vi "runtest client check.vi"(6 "Client IP or Domain Name (\"\")":string, 7 "POST (empty)":T4, 8 "error in (no error)":errorcluster, 9 "sxSequenceId":string, 10 "Username (\"\")":string, 11 "Connection Refnum":T5) -> (0 "error out":errorcluster, 3 "Connection Refnum":T5, 4 "User/Station":T1, 5 "POST out":T4)   [LabVIEW 2011]
uses:
  Summitek EXT/ODBC/SQL Controls/Connection Refnum.ctl
  ITK EXT/utils/keyedarr.llb/Keyed Array.ctl
  runtest User - Station.ctl
  server/database/Stations/Instruments/Instrument Record.ctl
  server/database/Stations/Step Associations/Step Association Record.ctl
  Summitek EXT/Miscellaneous/OGAB Version.ctl
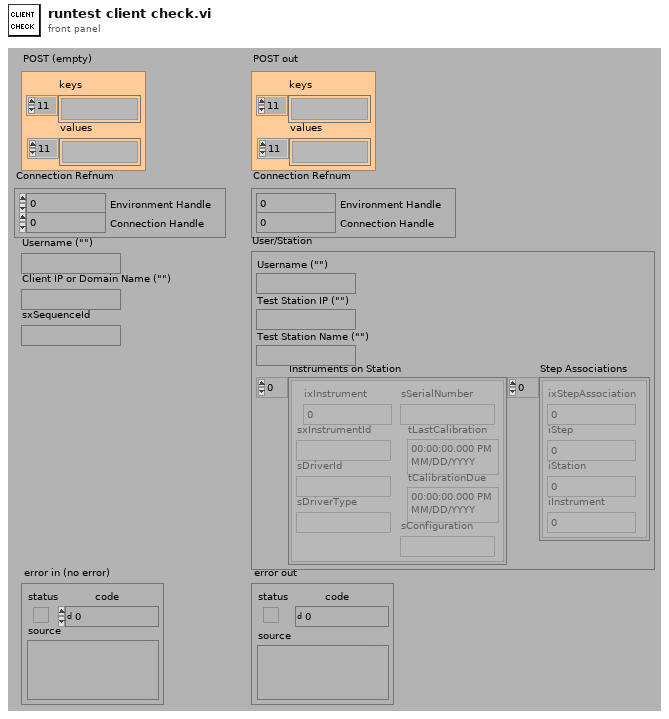
[diagram p1: front panel]
types:
  T1 = typedef "runtest User - Station.ctl" = cluster{"Username (\"\")":string, "Test Station IP (\"\")":string, "Test Station Name (\"\")":string, "Instruments on Station":T2[], "Step Associations":T3[]}
  T2 = typedef "Instrument Record.ctl" = cluster{"ixInstrument":i32, "sxInstrumentId":string, "sDriverId":string, "sDriverType":string, "sSerialNumber":string, "tLastCalibration":timestamp, "tCalibrationDue":timestamp, "sConfiguration":string}
  T3 = typedef "Step Association Record.ctl" = cluster{"ixStepAssociation":i32, "iStep":i32, "iStation":i32, "iInstrument":i32}
  T4 = typedef "Keyed Array.ctl" = cluster{"keys":string[], "values":string[]}
  T5 = typedef "Connection Refnum.ctl" = cluster{"Environment Handle":i32, "Connection Handle":i32}
  T6 = enum32{"invalid app kind", "Development System", "Run Time System", "Student Edition", "Embedded LabVIEW", "Evaluation", "Custom"}
  T7 = typedef "Station Record.ctl" = cluster{"ixStation":i32, "sxStationId":string, "sIP":string, "fVerified":bool}
  T8 = typedef "OGAB Version.ctl" = cluster{"Version":string, "Build Number":u32, "Build Date/Time":dbl}
  T9 = enum16{"Version 1 < Version 2", "Version 1 = Version 2", "Version 1 > Version 2"}
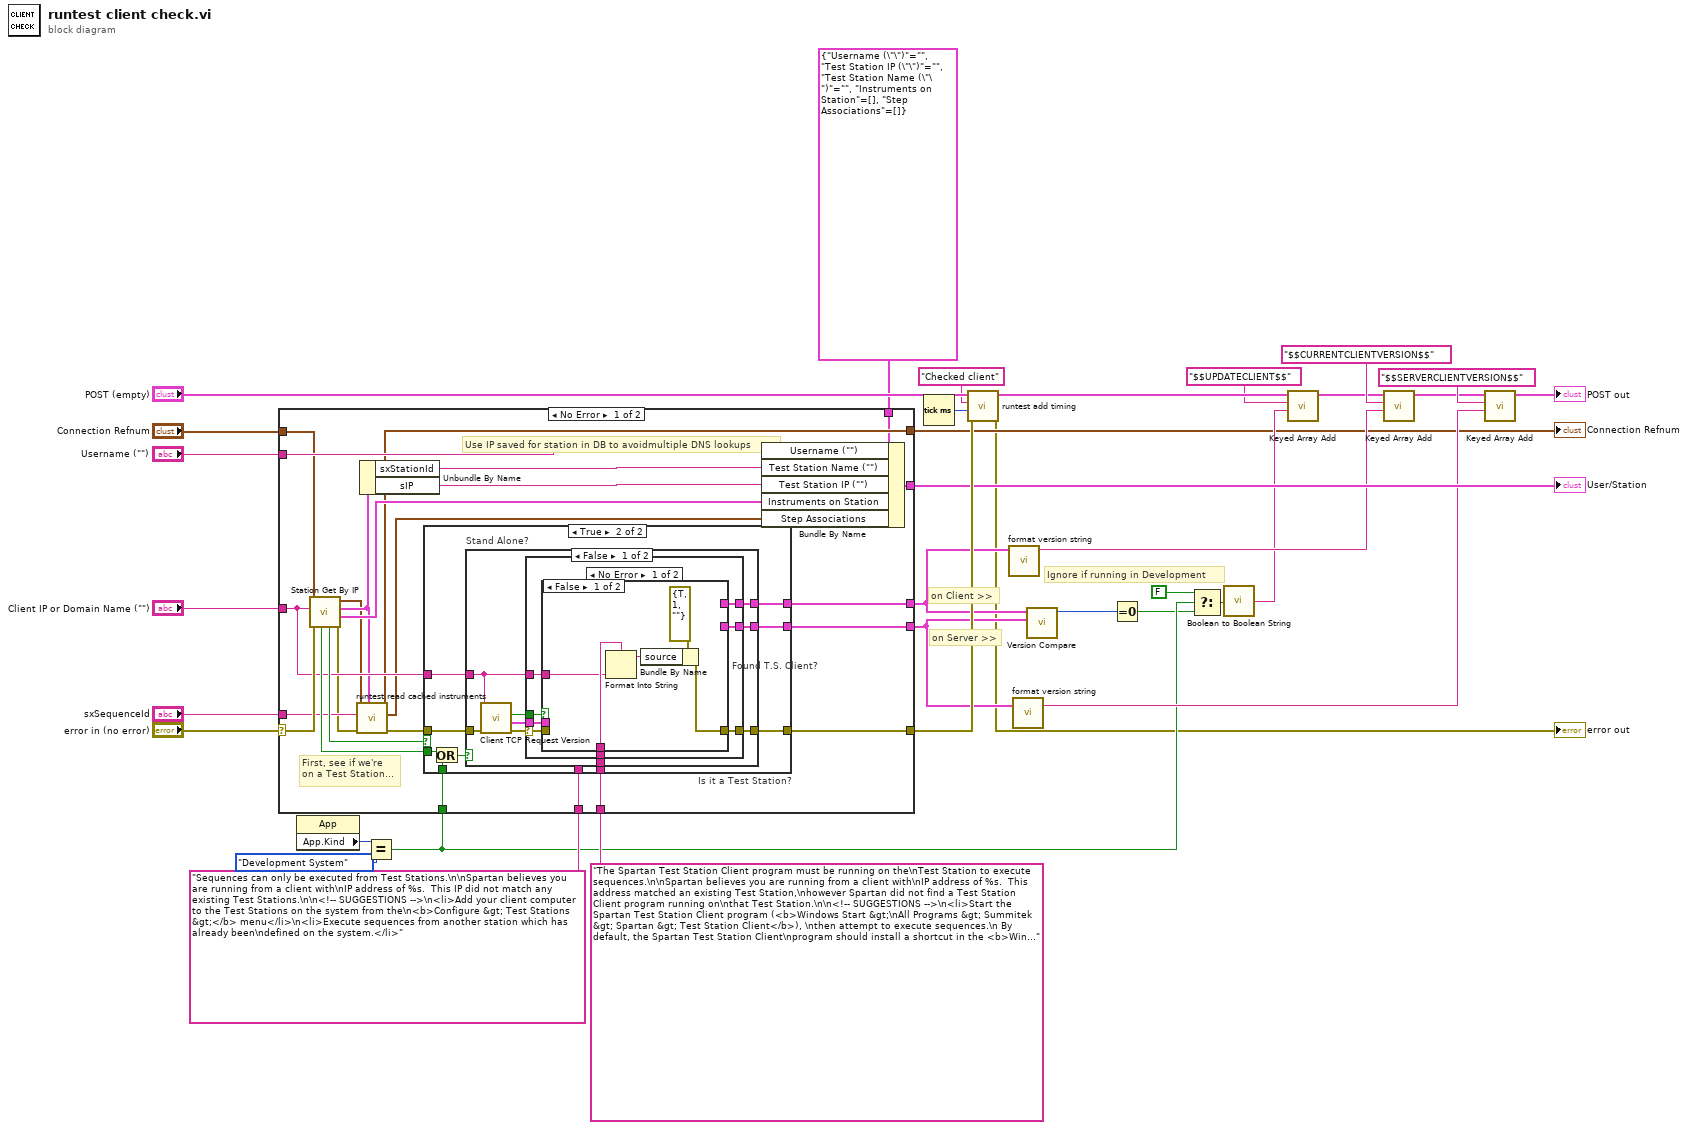
[diagram p0: block diagram]
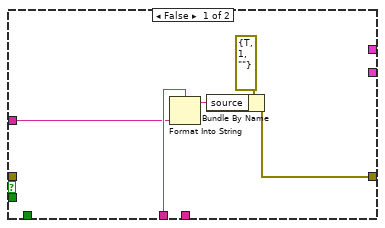
[diagram p2: hidden frame]
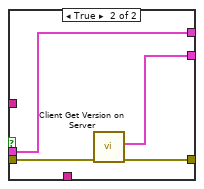
[diagram p3: hidden frame]
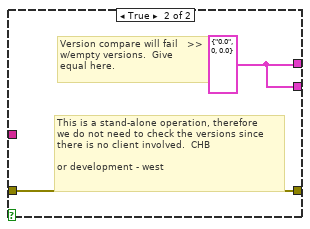
[diagram p5: hidden frame]
diagram:
  # "Ignore if running in Development"
  # "on Server >>"
  # "on Client >>"
  n1 = property class="App"() -> ("App.Kind"=w15:T6)  [unwired: 2 in, 2 out]
  n2 = Equal?(x=w15, y=T6."Development System") -> (x = y?=w11:bool)
  n3 = case shown="No Error" "error in (no error)" {
    selector: "error in (no error)" -> [w49 w103]
    tunnel: "Connection Refnum" -> [w48 w102]
    tunnel: [w39 w102] -> w4
    tunnel: "Client IP or Domain Name (\"\")" -> [w44 _]
    tunnel: [w58 w103] -> w28
    tunnel: "Sequences can only be executed from Test Stations.\n\nSpartan believes you are running from a client with\nIP address of %s.  This IP did not match any existing Test Stations.\n\n<!-- SUGGESTIONS -->\n<li>Add your client computer to the Test Stations on the system from the\n<b>Configure &gt; Test Stations &gt;</b> menu</li>\n<li>Execute sequences from another station which has already been\ndefined on the system.</li>" ("source") -> [w57 _]
    tunnel: "The Spartan Test Station Client program must be running on the\nTest Station to execute sequences.\n\nSpartan believes you are running from a client with\nIP address of %s.  This address matched an existing Test Station,\nhowever Spartan did not find a Test Station Client program running on\nthat Test Station.\n\n<!-- SUGGESTIONS -->\n<li>Start the Spartan Test Station Client program (<b>Windows Start &gt;\nAll Programs &gt; Summitek &gt; Spartan &gt; Test Station Client</b>), \nthen attempt to execute sequences.\n By default, the Spartan Test Station Client\nprogram should install a shortcut in the <b>Windows &gt; All Programs &gt;\nStartup</b> folder which would start the client automatically when you log in.</li>\n<li>By default Spartan uses TCP port 3363 to communicate with Test Station Clients.\nEnsure that this port is not blocked on either Spartan or the Client machine.</li>" ("source") -> [w56 _]
    tunnel: "Username (\"\")" -> [w55 _]
    tunnel: [w53 _] -> w26
    tunnel: [w52 _] -> w10
    tunnel: [w51 _] -> w9
    tunnel: w11 -> [w43 _]
    tunnel: "sxSequenceId" -> [w42 _]
    tunnel: T1 {"Username (\"\")"="", "Test Station IP (\"\")"="", "Test Station Name (\"\")"="", "Instruments on Station"=[], "Step Associations"=[]} ("User/Station") -> [w38 _]
    frame No Error {
      # "Use IP saved for station in DB to avoidmultiple DNS lookups"
      # "First, see if we're\non a Test Station..."
      n4 = call "Station Get By IP.vi"("error in (no error)"=w49, "IP or Name (\"\")"=w44, "Connection Refnum"=w48) -> ("error out"=w35:errorcluster, "Instruments on Station"=w47:T2[], "Station Record"=w41:T7, "Connection Refnum"=w40:T5, "Data Present?"=w45:bool, "Stand Alone?"=w46:bool)  [unwired: 1 in, 2 out]
      n5 = call "runtest read cached instruments.vi"("Station"=w41, "error in (no error)"=w35, "sxSequenceId"=w42, "Connection Refnum"=w40) -> ("error out"=w36:errorcluster, "Step Associations"=w37:T3[], "Connection Refnum"=w39:T5)  [unwired: 5 in]
      n6 = Unbundle By Name(w41) -> ("sxStationId"=w54:string, "sIP"=w50:string)
      n7 = case "Is it a Test Station?" shown="True" w45 {
        tunnel: w36 -> [_ w64]
        tunnel: w44 -> [w59 w65]
        tunnel: [w61 w72] -> w58
        tunnel: w57 -> [w63 _]
        tunnel: w56 -> [_ w71]
        tunnel: [_ w70] -> w52
        tunnel: [_ w69] -> w51
        tunnel: w46 -> [_ w67]
        tunnel: w43 -> [_ w68]
        frame False {
          n8 = Format Into String(format string=w63, w59) -> (resulting string=w60:string)  [unwired: 2 in, 1 out]
          n9 = Bundle By Name(cluster=errorcluster {"status"=TRUE, "code"=1, "source"=""} ("error out"), "source"=w60) -> (w61:errorcluster)
        }
        frame True {
          n10 = Or(x=w67, y=w68) -> (x .or. y?=w66:bool)
          n11 = case "Stand Alone?" shown="False" w66 {
            tunnel: w64 -> [w81 w101]
            tunnel: [w79 w101] -> w72
            tunnel: w71 -> [w78 _]
            tunnel: w65 -> [w77 _]
            tunnel: [w75 w100] -> w70
            tunnel: [w74 w100] -> w69
            frame False {
              n12 = call "Client TCP Request Version.vi"("error in (no error)"=w81, "Client IP"=w77) -> ("error out"=w73:errorcluster, "Client Version"=w76:T8, "Client Detected?"=w80:bool)  [unwired: 7 out]
              n13 = case shown="No Error" w73 {
                selector: w73 -> [w82 w99]
                tunnel: w80 -> [w89 _]
                tunnel: [w88 w99] -> w79
                tunnel: w78 -> [w87 _]
                tunnel: w77 -> [w86 _]
                tunnel: w76 -> [w85 _]
                tunnel: [w84 _] -> w75
                tunnel: [w83 _] -> w74
                frame No Error {
                  n14 = case "Found T.S. Client?" shown="False" w89 {
                    tunnel: w82 -> [_ w98]
                    tunnel: [w90 w97] -> w88
                    tunnel: w87 -> [w92 _]
                    tunnel: w86 -> [w91 _]
                    tunnel: w85 -> [_ w96]
                    tunnel: [_ w96] -> w84
                    tunnel: [_ w95] -> w83
                    frame False {
                      n15 = Format Into String(format string=w92, w91) -> (resulting string=w93:string)  [unwired: 2 in, 1 out]
                      n16 = Bundle By Name(cluster=errorcluster {"status"=TRUE, "code"=1, "source"=""} ("error out"), "source"=w93) -> (w90:errorcluster)
                    }
                    frame True {
                      n17 = call "Client Get Version on Server.vi"("error in (no error)"=w98) -> ("error out"=w97:errorcluster, "Version"=w95:T8)  [unwired: 9 out]
                    }
                  }
                }
                frame Error {
                }
              }
            }
            frame True {
              w100 = T8 {"Version"="0.0", "Build Number"=0, "Build Date/Time"=0.0} ("Client Version")
              # "Version compare will fail   >>\nw/empty versions.  Give\nequal here."
              # "This is a stand-alone operation, therefore\nwe do not need to check the versions since\nthere is no client involved.  CHB\n\nor development - west"
            }
          }
        }
      }
      n18 = Bundle By Name(cluster=w38, "Username (\"\")"=w55, "Test Station Name (\"\")"=w54, "Test Station IP (\"\")"=w50, "Instruments on Station"=w47, "Step Associations"=w37) -> (w53:T1)
    }
    frame Error {
    }
  }
  "Connection Refnum" <- w4
  "User/Station" <- w26
  n19 = Tick Count (ms)() -> (millisecond timer value=w27:u32)
  n20 = call "runtest add timing.vi"("error in (no error)"=w28, "Start Tick, ms (0)"=w27, "Function (\"\")"="Checked client", "POST (empty)"="POST (empty)") -> ("error out"=→"error out":errorcluster, "POST out"=w25:T4)  [unwired: 6 out]
  n21 = call "format version string.vi"("Version"=w10) -> ("Version String"=w20:string)  [unwired: 2 out]
  n22 = call "format version string.vi"("Version"=w9) -> ("Version String"=w19:string)  [unwired: 2 out]
  n23 = call "Version Compare.vi"("Version 1"=w10, "Version 2"=w9) -> ("Version Comparison"=w8:T9)  [unwired: 1 in, 5 out]
  n24 = Equal To 0?(x=w8) -> (x = 0?=w7:bool)
  n25 = Select(t=FALSE, s=w11, f=w7) -> (s? t:f=w12:bool)
  n26 = call "Boolean to Boolean String.vi"("Boolean"=w12) -> ("Boolean string"=w16:string)  [unwired: 1 in]
  n27 = call "Keyed Array Add.vi"("value"=w16, "key"="$$UPDATECLIENT$$", "array in"=w25) -> ("array out"=w18:T4)  [unwired: 1 in, 3 out]
  n28 = call "Keyed Array Add.vi"("value"=w20, "key"="$$CURRENTCLIENTVERSION$$", "array in"=w18) -> ("array out"=w21:T4)  [unwired: 1 in, 3 out]
  n29 = call "Keyed Array Add.vi"("value"=w19, "key"="$$SERVERCLIENTVERSION$$", "array in"=w21) -> ("array out"=→"POST out":T4)  [unwired: 1 in, 3 out]
